vi "CheckNetworkSettingsFile.vi"(8 "error in (no error)":errorcluster, 10 "hostname":string, 11 "upload path":path) -> (0 "error out":errorcluster, 1 "path":path, 2 "exists":bool, 3 "NetworkSettings":T1[](array[typedef]) {"IP Address Request Mode" items=["Static"=1, "DHCP/Link Local"=2, "Link-Local Only"=4, "DHCP Only"=8]; "Adapter Mode" items=["Disabled"=1, "TCP/IP Ethernet"=2, "Deterministic"=4, "EtherCAT"=8, "TCP/IP WLAN Connect"=32, "TCP/IP WLAN Create"=64]})   [LabVIEW 2017, in "USBDrive.lvlib"]
uses:
  <vilib>/addons/InsightCM/Devices/Shared/Common/USBDrive/USBDrive.lvlib
  <vilib>/addons/SystemInfoProcess/controls/NetworkAdapterSettings.ctl
  <vilib>/addons/SystemInfoProcess/SystemInfoProcess.lvlib
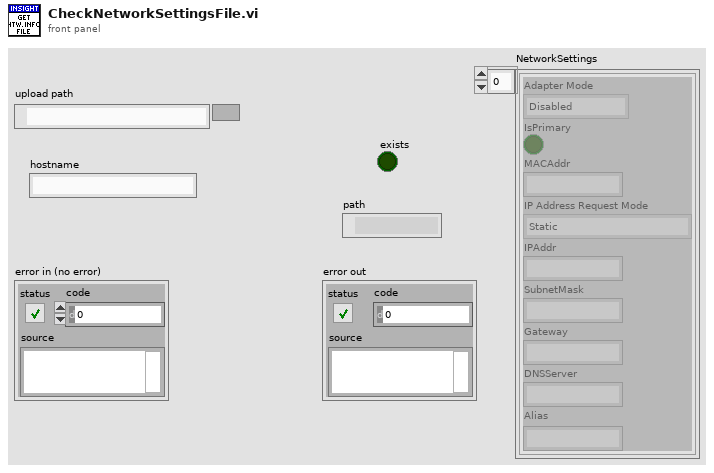
[diagram p1: front panel]
types:
  T1 = typedef "SystemInfoProcess.lvlib/NetworkAdapterSettings.ctl" = cluster{"Adapter Mode":u32, "IsPrimary":bool, "MACAddr":string, "IP Address Request Mode":u32, "IPAddr":string, "SubnetMask":string, "Gateway":string, "DNSServer":string, "Alias":string}
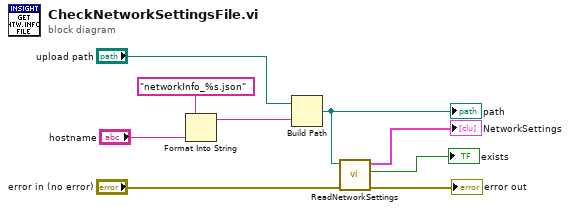
[diagram p0: block diagram]
diagram:
  n1 = Format Into String(format string="networkInfo_%s.json", "hostname") -> (resulting string=w4:string)  [unwired: 2 in, 1 out]
  n2 = Build Path(base path="upload path", name or relative path=w4) -> (appended path=w3:path)
  "path" <- w3
  n3 = call <vilib>:"ReadNetworkSettings.vi"("error in (no error)"="error in (no error)", "path"=w3) -> ("error out"=→"error out":errorcluster, "found"=→"exists":bool, "network settings"=→"NetworkSettings":T1[])  [unwired: 7 in]
